vi "Open (path).vi"(6 "SQLite Library Path":path, 7 "SQLite Connection type":refnum<class "Connection.lvclass">, 8 "error in (no error)":errorcluster, 10 "busy timeout (ms)":i32=5000, 11 "db file":path) -> (0 "error out":errorcluster, 3 "SQLite Connection out":refnum<class "Connection.lvclass">)   [LabVIEW 2011, in "SQLite.lvlib" / "Connection.lvclass"]
uses:
  Connection.lvclass
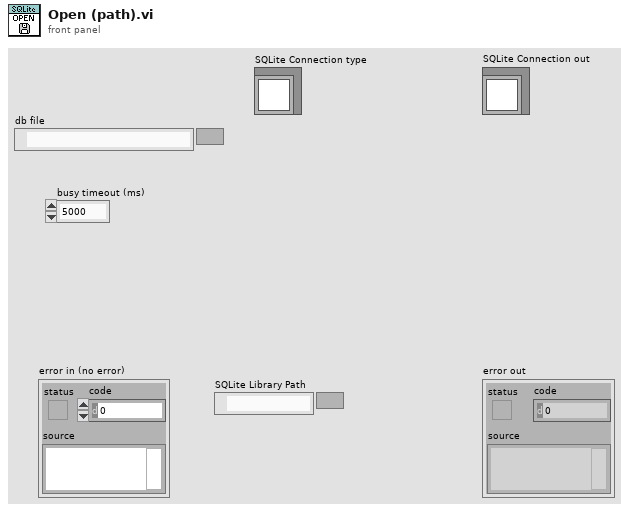
[diagram p1: front panel]
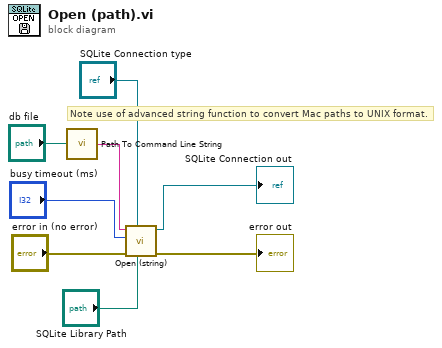
[diagram p0: block diagram]
diagram:
  # "Note use of advanced string function to convert Mac paths to UNIX format."
  n1 = call <vilib>:"Path To Command Line String.vi"("path"="db file") -> ("string"=w3:string)
  n2 = call "Open (string).vi"("SQLite Library Path"="SQLite Library Path", "SQLite Connection type"="SQLite Connection type", "error in (no error)"="error in (no error)", "busy timeout (ms)"="busy timeout (ms)", "db file"=w3) -> ("error out"=→"error out":errorcluster, "SQLite Connection out"=→"SQLite Connection out":refnum<class "Connection.lvclass">)  [unwired: 5 in]
